vi "FlowSensorSampleSensorLoop.vi"   [LabVIEW 2018]
uses:
  FlowSensorSampleSensorLoopData.ctl
  FlowSensorSampleSensorLoopStates.ctl
  FlowSensorSample.ctl
  FlowSensorErrorSample.ctl
  FlowSensorErrorCodes.ctl
  <vilib>/Platform/TimedLoop/XDataNode/timing_clust.ctl
  <vilib>/Platform/TimedLoop/XDataNode/nitl_modes.ctl
  <vilib>/Platform/TimedLoop/XDataNode/wakeup.ctl
  <vilib>/rvi/Emulation/niFpgaSctlEmulationGetInTimedLoop.vi
  <vilib>/rvi/Emulation/niFpgaEmulationReportErrorSimple.vi
  <vilib>/rvi/Emulation/niFpgaGetClockAttributes.vi
  <vilib>/rvi/Emulation/niFpgaCriticalErrorInLSC.vi
  <vilib>/rvi/Emulation/niFpgaEmulationIsFPGAContextNoSignature.vi
  <vilib>/rvi/errors/niFpgaSetErrorForExecOnDevCompSimple.vi
  <vilib>/rvi/eio/common/nirviEmuReportErrorAndStop.vi
  <vilib>/rvi/DataTransferAndStorage/Container/Common/niFpgaContainerGetUniqueNameForEmu.vi
  <vilib>/rvi/FIFO/Fifo_Resource/nirvififoEmulationSetSize.vi
  <vilib>/rvi/FIFO/Fifo_Resource/nirviFifoEmulationQueueMgr.vi
  <instcachedir>/0/nirviFifoEmulationQueueMgr_E5CAEC123FF24DC58D834DCA3CDAA9B5.lvgen/nirviFifoEmulationQueueMgr_E5CAEC123FF24DC58D834DCA3CDAA9B5_002.vi
  <vilib>/Utility/error.llb/Clear Errors.vi
  <vilib>/rvi/FIFO/Fifo_Resource/nirvififoEmulationCreateLock.vi
  <vilib>/rvi/Emulation/niFpgaProcessEmulError.vi
  <vilib>/rvi/FIFO/Fifo_Resource/nirvififoEmulationObtainLock.vi
  <vilib>/rvi/FIFO/Fifo_Resource/nirvififoEmulationReleaseLock.vi
  <vilib>/rvi/occurrence/nirviWaitOnOccurrenceBase.vi
  <vilib>/rvi/errors/nirviReportUnexpectedCaseInternalError.vi
  <vilib>/rvi/errors/nirviReportUnexpectedCaseInternalError (U32).vi
  <vilib>/rvi/FIFO/Fifo_Resource/nirvififoEmulationDetermineInputValidOut.vi
  <instcachedir>/0/nirviFifoEmulationQueueMgr_E5CAEC123FF24DC58D834DCA3CDAA9B5.lvgen/nirviFifoEmulationQueueMgr_E5CAEC123FF24DC58D834DCA3CDAA9B5_001.vi
  <instcachedir>/0/nirviFifoEmulationQueueMgr_E5CAEC123FF24DC58D834DCA3CDAA9B5.lvgen/nirviFifoEmulationQueueMgr_E5CAEC123FF24DC58D834DCA3CDAA9B5_004.vi
  <vilib>/rvi/Memory/Memory_Emulation/niFpgaMemoryEmulationCacheClearOnFirstRun.vi
  <vilib>/rvi/Memory/Memory_Emulation/nirvimemoryEmulationManagerCache_MakeExclusive.vi
  <vilib>/rvi/Memory/Memory_Emulation/niFpgaMemoryEmulationValidateCache.vi
  <vilib>/rvi/Memory/Memory_Emulation/nirvimemoryEmulationManagerCache_InsertValue.vi
  <vilib>/rvi/Memory/Memory_Emulation/nirvimemoryEmulationManagerCache_ReleaseExclusive.vi
  <vilib>/rvi/Memory/Memory_Emulation/nirvimemoryEmulationManagerCache_GetValue.vi
  <vilib>/rvi/Memory/Memory_Emulation/nirvimemoryEmulationManagerCache_SetValue.vi
  <instcachedir>/0/nirviFifoEmulationQueueMgr_E5CAEC123FF24DC58D834DCA3CDAA9B5.lvgen/nirviFifoEmulationQueueMgr_E5CAEC123FF24DC58D834DCA3CDAA9B5_028.vi
  <instcachedir>/0/nirviFifoEmulationQueueMgr_E5CAEC123FF24DC58D834DCA3CDAA9B5.lvgen/nirviFifoEmulationQueueMgr_E5CAEC123FF24DC58D834DCA3CDAA9B5_015.vi
  <vilib>/Platform/TimedLoop/XDataNode/XDataNode.xnode
  <vilib>/rvi/DataTransferAndStorage/Container/XNode/niFpgaContainer.xnode
  <vilib>/rvi/FIFO/Fifo_Resource/nirvififoEmulationRead.vi
  <vilib>/rvi/FIFO/Fifo_Resource/nirvififoEmulationWrite.vi
  <vilib>/rvi/DataTransferAndStorage/Register/Emulation/niFpgaRegisterEmulation.vi
  <vilib>/Platform/TimedLoop/XDataNode/XDNodeRunTimeDep.lvlib
types:
  T1 = typedef "FlowSensorSampleSensorLoopData.ctl" = cluster{"State":T2, "StateAfterRead":T2, "Timestamp":u64, "Timeout":i32, "U32":u32, "CRC":u16, "Exception":u8, "Sample":T3, "ErrorSample":T4}
  T2 = typedef "FlowSensorSampleSensorLoopStates.ctl" = enum16{"WaitForTrigger", "ClearRxFIFO", "WaitForClearComplete", "WriteAddress", "WriteFunction", "WriteStartAddress1", "WriteStartAddress0", "WriteAddressCount1", "WriteAddressCount0", "WriteCRC1", "WriteCRC0", "ReadAddress", "ReadFunction", "ReadByteCount", "StartSignalStrength", "EndSignalStrength", "StartFlowRate", "EndFlowRate", "StartNetTotalizer", "EndNetTotalizer", "StartPositiveTotalizer", "EndPositiveTotalizer", "StartNegativeTotalizer", "EndNegativeTotalizer", "StartTemperature1", "EndTemperature1", "StartTemperature2", "EndTemperature2", "ReadDataByte1", "ReadDataByte0", "ReadDataByte3", "ReadDataByte2", "ReadCRCByte0", "ReadCRCByte1", "CalculateCRC", "ValidateCRC", "PrepareSample", "MoveSample", "ReadExceptionCode", "ReadExceptionCRCByte0", "ReadExceptionCRCByte1", "CalculateExceptionCRC", "ValidateExceptionCRC", "ParseExceptionCode", "ResponseAddressError", "ResponseFunctionCodeError", "ResponseByteCountError", "ResponseCRCError", "ResponseUnknownError", "ResponseTimeoutError", "SensorReportsIllegalFunction", "SensorReportsIllegalDataAddress", "PrepareErrorCode", "MoveErrorCode"}
  T3 = typedef "FlowSensorSample.ctl" = cluster{"Timestamp":u64, "TxBytes":u64, "RxBytes":u64, "TxFrames":u64, "RxFrames":u64, "SignalStrength":u32, "FlowRate":u32, "NetTotalizer":u32, "PositiveTotalizer":u32, "NegativeTotalizer":u32, "Temperature1":u32, "Temperature2":u32}
  T4 = typedef "FlowSensorErrorSample.ctl" = cluster{"Timestamp":u64, "TxBytes":u64, "RxBytes":u64, "TxFrames":u64, "RxFrames":u64, "ErrorCode":T5}
  T5 = typedef "FlowSensorErrorCodes.ctl" = enum8{"None", "ResponseAddressError", "ResponseFunctionCodeError", "ResponseByteCountError", "ResponseCRCError", "ResponseUnknownError", "ResponseTimeoutError", "SensorReportsIllegalFunction", "SensorReportsIllegalDataAddress"}
  T6 = typedef "XDNodeRunTimeDep.lvlib/timing_clust.ctl" = cluster{"Expected End [f-1]":u64, "Actual End [f-1]":u64, "Finished Late? [f-1]":bool, "Expected End [i-1]":u64, "Actual End [i-1]":u64, "Finished Late? [i-1]":bool, "Expected Start [i]":u64, "Actual Start [i]":u64, "Expected Start [f]":u64, "Actual Start [f]":u64, "Source Name":string, "Structure Name":string, "Period":i64, "Deadline":i64, "Offset":i64, "Start":i64, "Priority":i32, "Timeout":i32, "Mode":T7, "Wakeup Reason":T8, "Error":errorcluster, "Source Type":string, "Secondary Source Type":string, "Global End Time":u64, "Global Start Time":u64, "Frame Duration":u64, "Iteration Duration":u64, "Assigned CPU":i32, "I/O Scan Engine Mode":u32}
  T7 = typedef "XDNodeRunTimeDep.lvlib/nitl_modes.ctl" = enum32{"No Change", "Process missed periods, maintain original phase", "Discard missed periods, maintain original phase", "Process missed periods, ignore original phase", "Discard missed periods, ignore original phase"}
  T8 = typedef "XDNodeRunTimeDep.lvlib/wakeup.ctl" = enum32{"Normal", "Aborted", "Asynchronous wakeup", "Timing source error", "Timed loop error", "Timeout"}
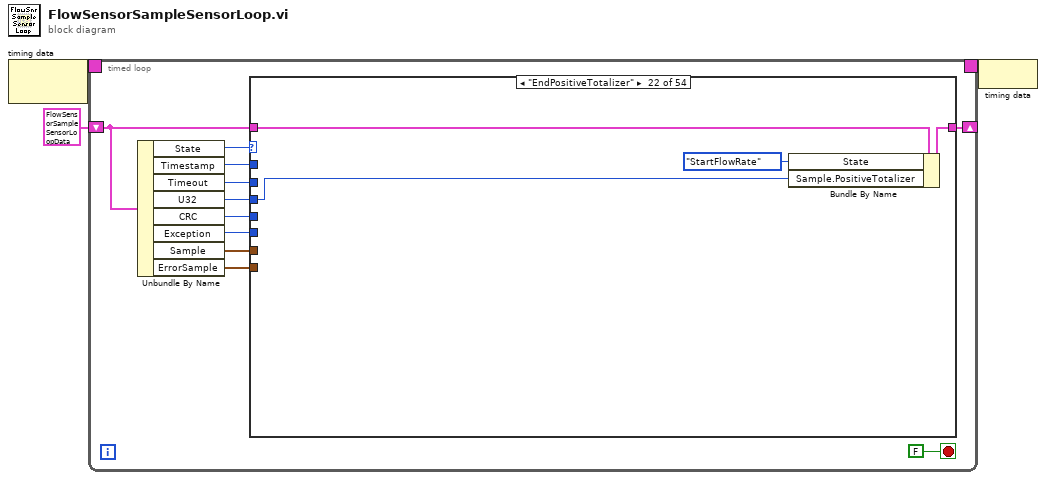
[diagram p0: block diagram]
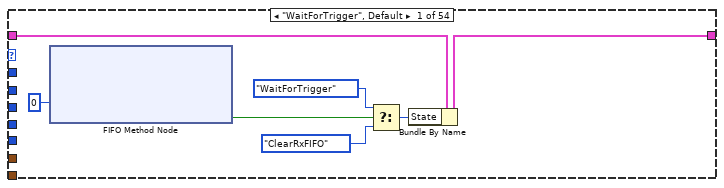
[diagram p2: hidden frame]
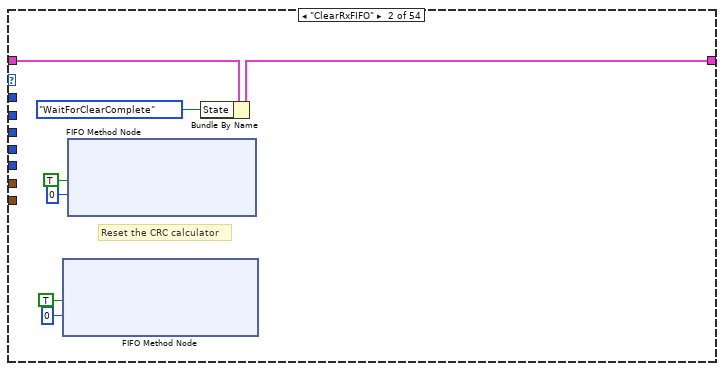
[diagram p3: hidden frame]
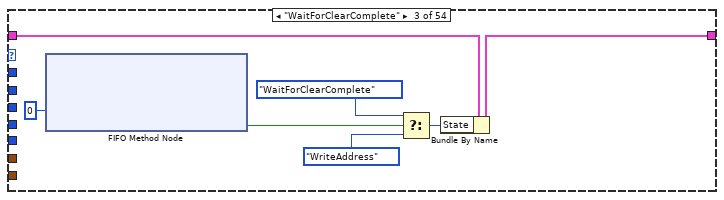
[diagram p4: hidden frame]
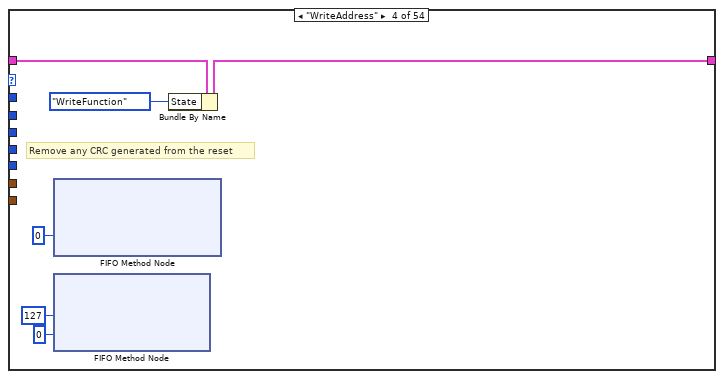
[diagram p5: hidden frame]
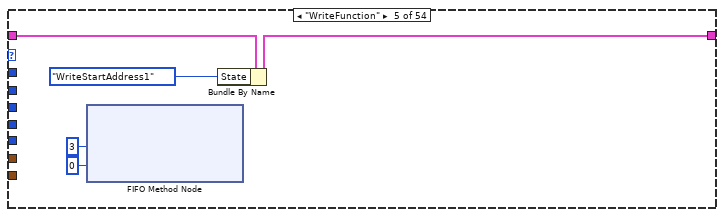
[diagram p6: hidden frame]
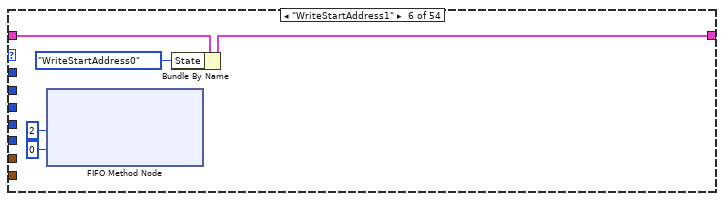
[diagram p7: hidden frame]
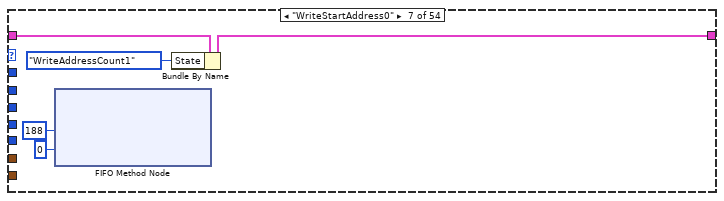
[diagram p8: hidden frame]
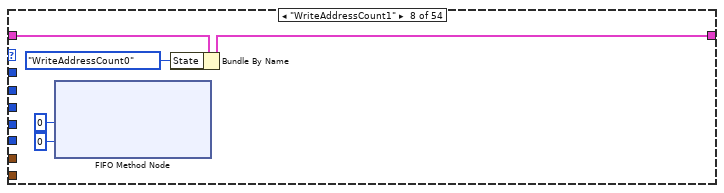
[diagram p9: hidden frame]
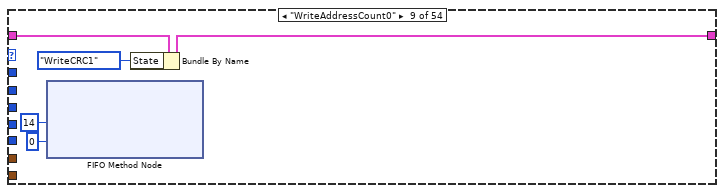
[diagram p10: hidden frame]
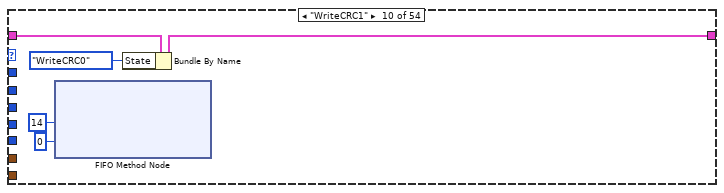
[diagram p11: hidden frame]
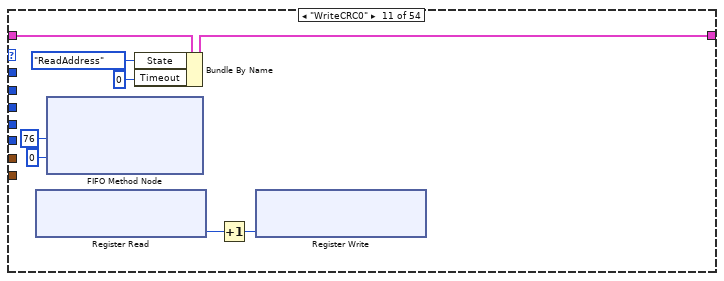
[diagram p12: hidden frame]
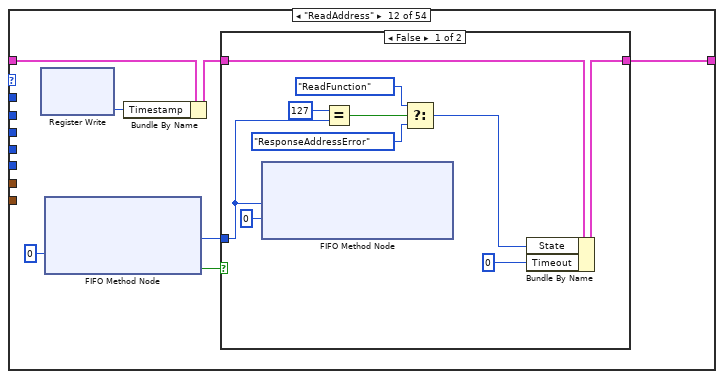
[diagram p13: hidden frame]
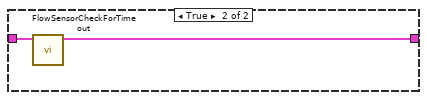
[diagram p14: hidden frame]
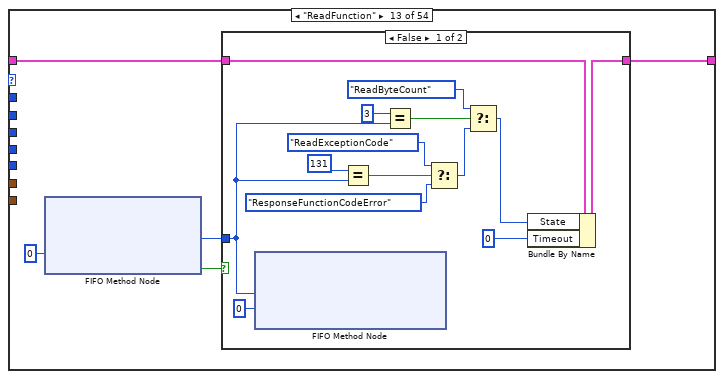
[diagram p15: hidden frame]
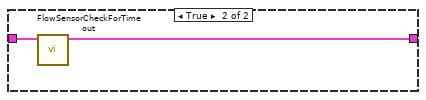
[diagram p16: hidden frame]
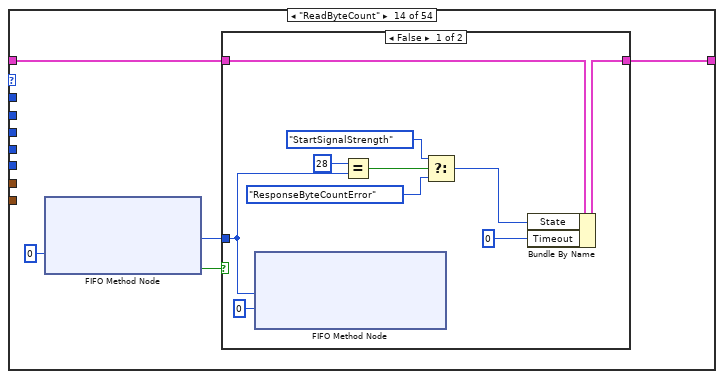
[diagram p17: hidden frame]
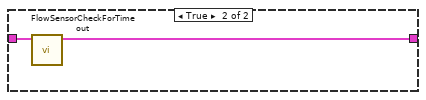
[diagram p18: hidden frame]
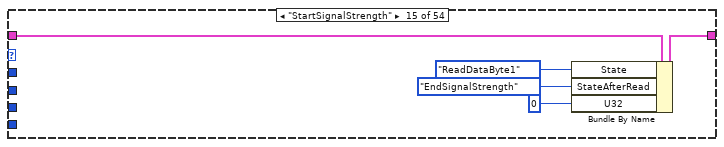
[diagram p19: hidden frame]
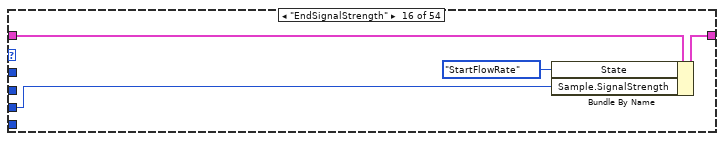
[diagram p20: hidden frame]
diagram:
  n1 = node-c288() -> (w3:T6)  [unwired: 1 in]
  n2 = timed-loop {
    timing: w3 -> [_]
    timing-out: [_] -> w2
    shift-right: [w13] -> _
    shift-left: T1 {"State"=enum."WaitForTrigger", "StateAfterRead"=enum."ClearRxFIFO", "Timestamp"=0, "Timeout"=0, "U32"=0, "CRC"=0, "Exception"=0, "Sample"={"Timestamp"=0, "TxBytes"=0, "RxBytes"=0, "TxFrames"=0, "RxFrames"=0, "SignalStrength"=0, "FlowRate"=0, "NetTotalizer"=0, "PositiveTotalizer"=0, "NegativeTotalizer"=0, "Temperature1"=0, "Temperature2"=0}, "ErrorSample"={"Timestamp"=0, "TxBytes"=0, "RxBytes"=0, "TxFrames"=0, "RxFrames"=0, "ErrorCode"=enum."None"}} ("InclinometerData") -> [w14]
    stop <- FALSE stop-if-true
    n3 = Unbundle By Name(w14) -> ("State"=w12:T2, "Timestamp"=w7:u64, "Timeout"=w11:i32, "U32"=w10:u32, "CRC"=w9:u16, "Exception"=w6:u8, "Sample"=w5:T3, "ErrorSample"=w4:T4)
    n4 = case shown="\"EndPositiveTotalizer\"" w12 {
      tunnel: w14 -> [w20 w27 w34 w40 w45 w50 w55 w60 w65 w70 w78 w82 w99 w120 w141 w145 w150 w154 w159 w163 w168 w172 w177 w181 w186 w190 w195 w199 w201 w224 w245 w266 w287 w307 w327 w332 w352 w357 w361 w382 w402 w422 w427 w447 w451 w455 w459 w463 w467 w471 w475 w479 w487 w492]
      tunnel: [w21 w28 w35 w41 w46 w51 w56 w61 w66 w71 w79 w83 w100 w121 w140 w144 w149 w153 w158 w162 w167 w171 w176 w180 w185 w189 w194 w198 w202 w225 w246 w267 w288 w308 w328 w333 w353 w358 w362 w383 w403 w423 w428 w448 w452 w456 w460 w464 w468 w472 w476 w480 w488 w493] -> w13
      tunnel: w11 -> [_ _ _ _ _ _ _ _ _ _ _ _ _ _ _ _ _ _ _ _ _ _ _ _ _ _ _ _ _ _ _ _ _ _ _ _ _ _ _ _ _ _ _ _ _ _ _ _ _ _ _ _ _ _]
      tunnel: w10 -> [_ _ _ _ _ _ _ _ _ _ _ _ _ _ _ w142 _ w151 _ w160 _ w169 _ w178 _ w187 _ w196 w200 w223 w244 w265 _ _ _ _ _ _ _ _ _ _ _ _ _ _ _ _ _ _ _ _ _ _]
      tunnel: w9 -> [_ _ _ _ _ _ _ _ _ _ _ _ _ _ _ _ _ _ _ _ _ _ _ _ _ _ _ _ _ _ _ _ w286 w306 _ w331 _ _ _ w381 w401 _ w426 _ _ _ _ _ _ _ _ _ _ _]
      tunnel: w7 -> [_ _ _ _ _ _ _ _ _ _ _ _ _ _ _ _ _ _ _ _ _ _ _ _ _ _ _ _ _ _ _ _ _ _ _ _ w351 _ _ _ _ _ _ _ _ _ _ _ _ _ _ _ w486 _]
      tunnel: w6 -> [_ _ _ _ _ _ _ _ _ _ _ _ _ _ _ _ _ _ _ _ _ _ _ _ _ _ _ _ _ _ _ _ _ _ _ _ _ _ _ _ _ _ _ w442 _ _ _ _ _ _ _ _ _ _]
      tunnel: w5 -> [_ _ _ _ _ _ _ _ _ _ _ _ _ _ _ _ _ _ _ _ _ _ _ _ _ _ _ _ _ _ _ _ _ _ _ _ _ w354 _ _ _ _ _ _ _ _ _ _ _ _ _ _ _ _]
      tunnel: w4 -> [_ _ _ _ _ _ _ _ _ _ _ _ _ _ _ _ _ _ _ _ _ _ _ _ _ _ _ _ _ _ _ _ _ _ _ _ _ _ _ _ _ _ _ _ _ _ _ _ _ _ _ _ _ w490]
      frame "WaitForTrigger", Default {
        n5 = xnode ("FIFO Method Node")("Timeout"=0) -> ("Timed Out?"=w15:bool)  [unwired: 1 in, 2 out]
        n6 = Select(t=FlowSensorSampleSensorLoopStates."WaitForTrigger" ("InclinometerState"), s=w15, f=FlowSensorSampleSensorLoopStates."ClearRxFIFO" ("InclinometerState")) -> (s? t:f=w17:T2)
        n7 = Bundle By Name(cluster=w20, "State"=w17) -> (w21:T1)
      }
      frame "ClearRxFIFO" {
        # "Reset the CRC calculator"
        n8 = xnode ("FIFO Method Node")("Element"=TRUE, "Timeout"=0) -> ()  [unwired: 1 in, 2 out]
        n9 = xnode ("FIFO Method Node")("Element"=TRUE, "Timeout"=0) -> ()  [unwired: 1 in, 2 out]
        n10 = Bundle By Name(cluster=w27, "State"=FlowSensorSampleSensorLoopStates."WaitForClearComplete" ("InclinometerState")) -> (w28:T1)
      }
      frame "WaitForClearComplete" {
        n11 = xnode ("FIFO Method Node")("Timeout"=0) -> ("Timed Out?"=w29:bool)  [unwired: 1 in, 2 out]
        n12 = Select(t=FlowSensorSampleSensorLoopStates."WaitForClearComplete", s=w29, f=FlowSensorSampleSensorLoopStates."WriteAddress" ("InclinometerState")) -> (s? t:f=w31:T2)
        n13 = Bundle By Name(cluster=w34, "State"=w31) -> (w35:T1)
      }
      frame "WriteAddress" {
        # "Remove any CRC generated from the reset"
        n14 = xnode ("FIFO Method Node")("Timeout"=0) -> ()  [unwired: 1 in, 3 out]
        n15 = xnode ("FIFO Method Node")("Element"=u8 127, "Timeout"=0) -> ()  [unwired: 1 in, 2 out]
        n16 = Bundle By Name(cluster=w40, "State"=FlowSensorSampleSensorLoopStates."WriteFunction" ("InclinometerState")) -> (w41:T1)
      }
      frame "WriteFunction" {
        n17 = xnode ("FIFO Method Node")("Element"=u8 3, "Timeout"=0) -> ()  [unwired: 1 in, 2 out]
        n18 = Bundle By Name(cluster=w45, "State"=FlowSensorSampleSensorLoopStates."WriteStartAddress1" ("InclinometerState")) -> (w46:T1)
      }
      frame "WriteStartAddress1" {
        n19 = xnode ("FIFO Method Node")("Element"=u8 2, "Timeout"=0) -> ()  [unwired: 1 in, 2 out]
        n20 = Bundle By Name(cluster=w50, "State"=FlowSensorSampleSensorLoopStates."WriteStartAddress0" ("InclinometerState")) -> (w51:T1)
      }
      frame "WriteStartAddress0" {
        n21 = xnode ("FIFO Method Node")("Element"=u8 188, "Timeout"=0) -> ()  [unwired: 1 in, 2 out]
        n22 = Bundle By Name(cluster=w55, "State"=FlowSensorSampleSensorLoopStates."WriteAddressCount1" ("InclinometerState")) -> (w56:T1)
      }
      frame "WriteAddressCount1" {
        n23 = xnode ("FIFO Method Node")("Element"=u8 0, "Timeout"=0) -> ()  [unwired: 1 in, 2 out]
        n24 = Bundle By Name(cluster=w60, "State"=FlowSensorSampleSensorLoopStates."WriteAddressCount0" ("InclinometerState")) -> (w61:T1)
      }
      frame "WriteAddressCount0" {
        n25 = xnode ("FIFO Method Node")("Element"=u8 14, "Timeout"=0) -> ()  [unwired: 1 in, 2 out]
        n26 = Bundle By Name(cluster=w65, "State"=FlowSensorSampleSensorLoopStates."WriteCRC1" ("InclinometerState")) -> (w66:T1)
      }
      frame "WriteCRC1" {
        n27 = xnode ("FIFO Method Node")("Element"=u8 14, "Timeout"=0) -> ()  [unwired: 1 in, 2 out]
        n28 = Bundle By Name(cluster=w70, "State"=FlowSensorSampleSensorLoopStates."WriteCRC0" ("InclinometerState")) -> (w71:T1)
      }
      frame "WriteCRC0" {
        n29 = xnode ("Register Read")() -> ("Data"=w73:u64)  [unwired: 1 in, 1 out]
        n30 = xnode ("FIFO Method Node")("Element"=u8 76, "Timeout"=0) -> ()  [unwired: 1 in, 2 out]
        n31 = Bundle By Name(cluster=w78, "State"=FlowSensorSampleSensorLoopStates."ReadAddress" ("InclinometerState"), "Timeout"=0) -> (w79:T1)
        n32 = Increment(x=w73) -> (x+1=w72:u64)
        n33 = xnode ("Register Write")("Data"=w72) -> ()  [unwired: 1 in, 1 out]
      }
      frame "ReadAddress" {
        n34 = xnode "Register Write"() -> ("Data"=w80:u64)  [unwired: 1 in, 1 out]
        n35 = xnode ("FIFO Method Node")("Timeout"=0) -> ("Element"=w84:u8, "Timed Out?"=w85:bool)  [unwired: 1 in, 1 out]
        n36 = Bundle By Name(cluster=w82, "Timestamp"=w80) -> (w81:T1)
        n37 = case shown="False" w85 {
          tunnel: w84 -> [w93 _]
          tunnel: [w95 w97] -> w83
          tunnel: w81 -> [w96 w98]
          frame False {
            n38 = xnode ("FIFO Method Node")("Element"=w93, "Timeout"=0) -> ()  [unwired: 1 in, 2 out]
            n39 = Equal?(x=u8 127, y=w93) -> (x = y?=w91:bool)
            n40 = Select(t=FlowSensorSampleSensorLoopStates."ReadFunction" ("InclinometerState"), s=w91, f=FlowSensorSampleSensorLoopStates."ResponseAddressError" ("InclinometerState")) -> (s? t:f=w88:T2)
            n41 = Bundle By Name(cluster=w96, "State"=w88, "Timeout"=0) -> (w95:T1)
          }
          frame True {
            n42 = call "FlowSensorCheckForTimeout.vi"("FlowSensorSampleSensorLoopData in"=w98) -> ("FlowSensorSampleSensorLoopData out"=w97:T1)  [unwired: 10 in]
          }
        }
      }
      frame "ReadFunction" {
        n43 = xnode ("FIFO Method Node")("Timeout"=0) -> ("Element"=w101:u8, "Timed Out?"=w102:bool)  [unwired: 1 in, 1 out]
        n44 = case shown="False" w102 {
          tunnel: w101 -> [w109 _]
          tunnel: [w116 w118] -> w100
          tunnel: w99 -> [w117 w119]
          frame False {
            n45 = xnode ("FIFO Method Node")("Element"=w109, "Timeout"=0) -> ()  [unwired: 1 in, 2 out]
            n46 = Equal?(x=u8 131, y=w109) -> (x = y?=w108:bool)
            n47 = Equal?(x=u8 3, y=w109) -> (x = y?=w113:bool)
            n48 = Select(t=FlowSensorSampleSensorLoopStates."ReadExceptionCode" ("InclinometerState"), s=w108, f=FlowSensorSampleSensorLoopStates."ResponseFunctionCodeError" ("InclinometerState")) -> (s? t:f=w111:T2)
            n49 = Select(t=FlowSensorSampleSensorLoopStates."ReadByteCount" ("InclinometerState"), s=w113, f=w111) -> (s? t:f=w105:T2)
            n50 = Bundle By Name(cluster=w117, "State"=w105, "Timeout"=0) -> (w116:T1)
          }
          frame True {
            n51 = call "FlowSensorCheckForTimeout.vi"("FlowSensorSampleSensorLoopData in"=w119) -> ("FlowSensorSampleSensorLoopData out"=w118:T1)  [unwired: 10 in]
          }
        }
      }
      frame "ReadByteCount" {
        n52 = xnode ("FIFO Method Node")("Timeout"=0) -> ("Element"=w122:u8, "Timed Out?"=w123:bool)  [unwired: 1 in, 1 out]
        n53 = case shown="False" w123 {
          tunnel: w122 -> [w131 _]
          tunnel: [w133 w135] -> w121
          tunnel: w120 -> [w134 w136]
          frame False {
            n54 = xnode ("FIFO Method Node")("Element"=w131, "Timeout"=0) -> ()  [unwired: 1 in, 2 out]
            n55 = Equal?(x=u8 28, y=w131) -> (x = y?=w129:bool)
            n56 = Select(t=FlowSensorSampleSensorLoopStates."StartSignalStrength" ("InclinometerState"), s=w129, f=FlowSensorSampleSensorLoopStates."ResponseByteCountError" ("InclinometerState")) -> (s? t:f=w126:T2)
            n57 = Bundle By Name(cluster=w134, "State"=w126, "Timeout"=0) -> (w133:T1)
          }
          frame True {
            n58 = call "FlowSensorCheckForTimeout.vi"("FlowSensorSampleSensorLoopData in"=w136) -> ("FlowSensorSampleSensorLoopData out"=w135:T1)  [unwired: 10 in]
          }
        }
      }
      frame "StartSignalStrength" {
        n59 = Bundle By Name(cluster=w141, "State"=FlowSensorSampleSensorLoopStates."ReadDataByte1", "StateAfterRead"=FlowSensorSampleSensorLoopStates."EndSignalStrength", "U32"=u32 0) -> (w140:T1)
      }
      frame "EndSignalStrength" {
        n60 = Bundle By Name(cluster=w145, "State"=FlowSensorSampleSensorLoopStates."StartFlowRate", "Sample.SignalStrength"=w142) -> (w144:T1)
      }
      frame "StartFlowRate" {
        n61 = Bundle By Name(cluster=w150, "State"=FlowSensorSampleSensorLoopStates."ReadDataByte1", "StateAfterRead"=FlowSensorSampleSensorLoopStates."EndFlowRate", "U32"=u32 0) -> (w149:T1)
      }
      frame "EndFlowRate" {
        n62 = Bundle By Name(cluster=w154, "State"=FlowSensorSampleSensorLoopStates."StartNetTotalizer", "Sample.FlowRate"=w151) -> (w153:T1)
      }
      frame "StartNetTotalizer" {
        n63 = Bundle By Name(cluster=w159, "State"=FlowSensorSampleSensorLoopStates."ReadDataByte1", "StateAfterRead"=FlowSensorSampleSensorLoopStates."EndNetTotalizer", "U32"=u32 0) -> (w158:T1)
      }
      frame "EndNetTotalizer" {
        n64 = Bundle By Name(cluster=w163, "State"=FlowSensorSampleSensorLoopStates."StartPositiveTotalizer", "Sample.NetTotalizer"=w160) -> (w162:T1)
      }
      frame "StartPositiveTotalizer" {
        n65 = Bundle By Name(cluster=w168, "State"=FlowSensorSampleSensorLoopStates."ReadDataByte1", "StateAfterRead"=FlowSensorSampleSensorLoopStates."EndPositiveTotalizer", "U32"=u32 0) -> (w167:T1)
      }
      frame "EndPositiveTotalizer" {
        n66 = Bundle By Name(cluster=w172, "State"=FlowSensorSampleSensorLoopStates."StartFlowRate", "Sample.PositiveTotalizer"=w169) -> (w171:T1)
      }
      frame "StartNegativeTotalizer" {
        n67 = Bundle By Name(cluster=w177, "State"=FlowSensorSampleSensorLoopStates."ReadDataByte1", "StateAfterRead"=FlowSensorSampleSensorLoopStates."EndNegativeTotalizer", "U32"=u32 0) -> (w176:T1)
      }
      frame "EndNegativeTotalizer" {
        n68 = Bundle By Name(cluster=w181, "State"=FlowSensorSampleSensorLoopStates."StartTemperature1", "Sample.NegativeTotalizer"=w178) -> (w180:T1)
      }
      frame "StartTemperature1" {
        n69 = Bundle By Name(cluster=w186, "State"=FlowSensorSampleSensorLoopStates."ReadDataByte1", "StateAfterRead"=FlowSensorSampleSensorLoopStates."EndTemperature1", "U32"=u32 0) -> (w185:T1)
      }
      frame "EndTemperature1" {
        n70 = Bundle By Name(cluster=w190, "State"=FlowSensorSampleSensorLoopStates."StartTemperature2", "Sample.Temperature1"=w187) -> (w189:T1)
      }
      frame "StartTemperature2" {
        n71 = Bundle By Name(cluster=w195, "State"=FlowSensorSampleSensorLoopStates."ReadDataByte1", "StateAfterRead"=FlowSensorSampleSensorLoopStates."EndTemperature2", "U32"=u32 0) -> (w194:T1)
      }
      frame "EndTemperature2" {
        n72 = Bundle By Name(cluster=w199, "State"=FlowSensorSampleSensorLoopStates."ReadCRCByte0", "Sample.Temperature2"=w196) -> (w198:T1)
      }
      frame "ReadDataByte1" {
        n73 = xnode ("FIFO Method Node")("Timeout"=0) -> ("Element"=w203:u8, "Timed Out?"=w204:bool)  [unwired: 1 in, 1 out]
        n74 = case shown="False" w204 {
          tunnel: w203 -> [w209 _]
          tunnel: [w217 w219] -> w202
          tunnel: w201 -> [w218 w220]
          tunnel: w200 -> [w213 _]
          frame False {
            n75 = To Unsigned Long Integer(number=w209) -> (unsigned 32bit integer=w208:u32)
            n76 = xnode ("FIFO Method Node")("Element"=w209, "Timeout"=0) -> ()  [unwired: 1 in, 2 out]
            n77 = Logical Shift(y=i16 8, x=w208) -> (x << y=w211:u32)
            n78 = And(x=u32 4294902015, y=w213) -> (x .and. y?=w210:u32)
            n79 = Or(x=w210, y=w211) -> (x .or. y?=w207:u32)
            n80 = Bundle By Name(cluster=w218, "State"=FlowSensorSampleSensorLoopStates."ReadDataByte0" ("InclinometerState"), "U32"=w207, "Timeout"=0) -> (w217:T1)
          }
          frame True {
            n81 = call "FlowSensorCheckForTimeout.vi"("FlowSensorSampleSensorLoopData in"=w220) -> ("FlowSensorSampleSensorLoopData out"=w219:T1)  [unwired: 10 in]
          }
        }
      }
      frame "ReadDataByte0" {
        n82 = xnode ("FIFO Method Node")("Timeout"=0) -> ("Element"=w226:u8, "Timed Out?"=w222:bool)  [unwired: 1 in, 1 out]
        n83 = case shown="False" w222 {
          tunnel: w226 -> [w227 _]
          tunnel: [w238 w240] -> w225
          tunnel: w224 -> [w239 w241]
          tunnel: w223 -> [w235 _]
          frame False {
            n84 = To Unsigned Long Integer(number=w227) -> (unsigned 32bit integer=w231:u32)
            n85 = xnode ("FIFO Method Node")("Element"=w227, "Timeout"=0) -> ()  [unwired: 1 in, 2 out]
            n86 = Logical Shift(y=i16 0, x=w231) -> (x << y=w233:u32)
            n87 = And(x=u32 4294967040, y=w235) -> (x .and. y?=w232:u32)
            n88 = Or(x=w232, y=w233) -> (x .or. y?=w230:u32)
            n89 = Bundle By Name(cluster=w239, "State"=FlowSensorSampleSensorLoopStates."ReadDataByte3" ("InclinometerState"), "U32"=w230, "Timeout"=0) -> (w238:T1)
          }
          frame True {
            n90 = call "FlowSensorCheckForTimeout.vi"("FlowSensorSampleSensorLoopData in"=w241) -> ("FlowSensorSampleSensorLoopData out"=w240:T1)  [unwired: 10 in]
          }
        }
      }
      frame "ReadDataByte3" {
        n91 = xnode ("FIFO Method Node")("Timeout"=0) -> ("Element"=w247:u8, "Timed Out?"=w242:bool)  [unwired: 1 in, 1 out]
        n92 = case shown="False" w242 {
          tunnel: w247 -> [w249 _]
          tunnel: [w259 w261] -> w246
          tunnel: w245 -> [w260 w262]
          tunnel: w244 -> [w256 _]
          frame False {
            n93 = To Unsigned Long Integer(number=w249) -> (unsigned 32bit integer=w252:u32)
            n94 = xnode ("FIFO Method Node")("Element"=w249, "Timeout"=0) -> ()  [unwired: 1 in, 2 out]
            n95 = Logical Shift(y=i16 24, x=w252) -> (x << y=w254:u32)
            n96 = And(x=u32 16777215, y=w256) -> (x .and. y?=w253:u32)
            n97 = Or(x=w253, y=w254) -> (x .or. y?=w251:u32)
            n98 = Bundle By Name(cluster=w260, "State"=FlowSensorSampleSensorLoopStates."ReadDataByte2" ("InclinometerState"), "U32"=w251, "Timeout"=0) -> (w259:T1)
          }
          frame True {
            n99 = call "FlowSensorCheckForTimeout.vi"("FlowSensorSampleSensorLoopData in"=w262) -> ("FlowSensorSampleSensorLoopData out"=w261:T1)  [unwired: 10 in]
          }
        }
      }
      frame "ReadDataByte2" {
        n100 = xnode ("FIFO Method Node")("Timeout"=0) -> ("Element"=w268:u8, "Timed Out?"=w263:bool)  [unwired: 1 in, 1 out]
        n101 = case shown="False" w263 {
          tunnel: w268 -> [w271 _]
          tunnel: [w281 w282] -> w267
          tunnel: w266 -> [w270 w283]
          tunnel: w265 -> [w279 _]
          frame False {
            n102 = To Unsigned Long Integer(number=w271) -> (unsigned 32bit integer=w275:u32)
            n103 = xnode ("FIFO Method Node")("Element"=w271, "Timeout"=0) -> ()  [unwired: 1 in, 2 out]
            n104 = Logical Shift(y=i16 16, x=w275) -> (x << y=w277:u32)
            n105 = And(x=u32 4278255615, y=w279) -> (x .and. y?=w276:u32)
            n106 = Or(x=w276, y=w277) -> (x .or. y?=w274:u32)
            n107 = Unbundle By Name(w270) -> ("StateAfterRead"=w269:T2)
            n108 = Bundle By Name(cluster=w270, "State"=w269, "U32"=w274, "Timeout"=0) -> (w281:T1)
          }
          frame True {
            n109 = call "FlowSensorCheckForTimeout.vi"("FlowSensorSampleSensorLoopData in"=w283) -> ("FlowSensorSampleSensorLoopData out"=w282:T1)  [unwired: 10 in]
          }
        }
      }
      frame "ReadCRCByte0" {
        n110 = xnode ("FIFO Method Node")("Timeout"=0) -> ("Element"=w289:u8, "Timed Out?"=w284:bool)  [unwired: 1 in, 1 out]
        n111 = case shown="False" w284 {
          tunnel: w289 -> [w290 _]
          tunnel: [w300 w302] -> w288
          tunnel: w287 -> [w301 w303]
          tunnel: w286 -> [w292 _]
          frame False {
            n112 = To Unsigned Word Integer(number=w290) -> (unsigned 16bit integer=w294:u16)
            n113 = Logical Shift(y=i16 0, x=w294) -> (x << y=w296:u16)
            n114 = And(x=u16 65280, y=w292) -> (x .and. y?=w295:u16)
            n115 = Or(x=w295, y=w296) -> (x .or. y?=w293:u16)
            n116 = Bundle By Name(cluster=w301, "State"=FlowSensorSampleSensorLoopStates."ReadCRCByte1" ("InclinometerState"), "CRC"=w293, "Timeout"=0) -> (w300:T1)
          }
          frame True {
            n117 = call "FlowSensorCheckForTimeout.vi"("FlowSensorSampleSensorLoopData in"=w303) -> ("FlowSensorSampleSensorLoopData out"=w302:T1)  [unwired: 10 in]
          }
        }
      }
      frame "ReadCRCByte1" {
        n118 = xnode ("FIFO Method Node")("Timeout"=0) -> ("Element"=w309:u8, "Timed Out?"=w304:bool)  [unwired: 1 in, 1 out]
        n119 = case shown="False" w304 {
          tunnel: w309 -> [w310 _]
          tunnel: [w320 w322] -> w308
          tunnel: w307 -> [w321 w323]
          tunnel: w306 -> [w312 _]
          frame False {
            n120 = To Unsigned Word Integer(number=w310) -> (unsigned 16bit integer=w314:u16)
            n121 = Logical Shift(y=i16 8, x=w314) -> (x << y=w316:u16)
            n122 = And(x=u16 255, y=w312) -> (x .and. y?=w315:u16)
            n123 = Or(x=w315, y=w316) -> (x .or. y?=w313:u16)
            n124 = Bundle By Name(cluster=w321, "State"=FlowSensorSampleSensorLoopStates."CalculateCRC" ("InclinometerState"), "CRC"=w313, "Timeout"=0) -> (w320:T1)
          }
          frame True {
            n125 = call "FlowSensorCheckForTimeout.vi"("FlowSensorSampleSensorLoopData in"=w323) -> ("FlowSensorSampleSensorLoopData out"=w322:T1)  [unwired: 10 in]
          }
        }
      }
      frame "CalculateCRC" {
        n126 = xnode ("FIFO Method Node")("Element"=TRUE, "Timeout"=0) -> ()  [unwired: 1 in, 2 out]
        n127 = Bundle By Name(cluster=w327, "State"=FlowSensorSampleSensorLoopStates."ValidateCRC" ("InclinometerState")) -> (w328:T1)
      }
      frame "ValidateCRC" {
        n128 = xnode ("FIFO Method Node")("Timeout"=0) -> ("Element"=w334:u16, "Timed Out?"=w329:bool)  [unwired: 1 in, 1 out]
        n129 = case shown="False" w329 {
          tunnel: w334 -> [w335 _]
          tunnel: [w343 w345] -> w333
          tunnel: w332 -> [w344 w345]
          tunnel: w331 -> [w338 _]
          frame False {
            n130 = xnode ("Register Read")() -> ("Data"=w337:u64)  [unwired: 1 in, 1 out]
            n131 = Equal?(x=w338, y=w335) -> (x = y?=w342:bool)
            n132 = Select(t=FlowSensorSampleSensorLoopStates."PrepareSample" ("InclinometerState"), s=w342, f=FlowSensorSampleSensorLoopStates."ResponseCRCError" ("InclinometerState")) -> (s? t:f=w339:T2)
            n133 = Increment(x=w337) -> (x+1=w336:u64)
            n134 = xnode ("Register Write")("Data"=w336) -> ()  [unwired: 1 in, 1 out]
            n135 = Bundle By Name(cluster=w344, "State"=w339) -> (w343:T1)
          }
          frame True {
          }
        }
      }
      frame "PrepareSample" {
        n136 = xnode ("Register Read")() -> ("Data"=w349:u64)  [unwired: 1 in, 1 out]
        n137 = xnode ("Register Read")() -> ("Data"=w348:u64)  [unwired: 1 in, 1 out]
        n138 = xnode ("Register Read")() -> ("Data"=w347:u64)  [unwired: 1 in, 1 out]
        n139 = xnode ("Register Read")() -> ("Data"=w346:u64)  [unwired: 1 in, 1 out]
        n140 = Bundle By Name(cluster=w352, "State"=FlowSensorSampleSensorLoopStates."MoveSample", "Sample.Timestamp"=w351, "Sample.TxBytes"=w349, "Sample.RxBytes"=w348, "Sample.TxFrames"=w347, "Sample.RxFrames"=w346) -> (w353:T1)
      }
      frame "MoveSample" {
        n141 = xnode ("FIFO Method Node")("Element"=w354, "Timeout"=0) -> ()  [unwired: 1 in, 2 out]
        n142 = Bundle By Name(cluster=w357, "State"=FlowSensorSampleSensorLoopStates."WaitForTrigger") -> (w358:T1)
      }
      frame "ReadExceptionCode" {
        n143 = xnode ("FIFO Method Node")("Timeout"=0) -> ("Element"=w363:u8, "Timed Out?"=w359:bool)  [unwired: 1 in, 1 out]
        n144 = case shown="False" w359 {
          tunnel: w363 -> [w364 _]
          tunnel: [w375 w377] -> w362
          tunnel: w361 -> [w376 w378]
          frame False {
            n145 = xnode ("FIFO Method Node")("Element"=w364, "Timeout"=0) -> ()  [unwired: 1 in, 2 out]
            n146 = Equal?(x=u8 1, y=w364) -> (x = y?=w368:bool)
            n147 = Equal?(x=u8 2, y=w364) -> (x = y?=w367:bool)
            n148 = Or(x=w368, y=w367) -> (x .or. y?=w366:bool)
            n149 = Select(t=FlowSensorSampleSensorLoopStates."ReadExceptionCRCByte0" ("InclinometerState"), s=w366, f=FlowSensorSampleSensorLoopStates."ResponseUnknownError" ("InclinometerState")) -> (s? t:f=w371:T2)
            n150 = Bundle By Name(cluster=w376, "State"=w371, "Timeout"=0, "Exception"=w364) -> (w375:T1)
          }
          frame True {
            n151 = call "FlowSensorCheckForTimeout.vi"("FlowSensorSampleSensorLoopData in"=w378) -> ("FlowSensorSampleSensorLoopData out"=w377:T1)  [unwired: 10 in]
          }
        }
      }
      frame "ReadExceptionCRCByte0" {
        n152 = xnode ("FIFO Method Node")("Timeout"=0) -> ("Element"=w384:u8, "Timed Out?"=w379:bool)  [unwired: 1 in, 1 out]
        n153 = case shown="False" w379 {
          tunnel: w384 -> [w385 _]
          tunnel: [w395 w397] -> w383
          tunnel: w382 -> [w396 w398]
          tunnel: w381 -> [w387 _]
          frame False {
            n154 = To Unsigned Word Integer(number=w385) -> (unsigned 16bit integer=w389:u16)
            n155 = Logical Shift(y=i16 0, x=w389) -> (x << y=w391:u16)
            n156 = And(x=u16 65280, y=w387) -> (x .and. y?=w390:u16)
            n157 = Or(x=w390, y=w391) -> (x .or. y?=w388:u16)
            n158 = Bundle By Name(cluster=w396, "State"=FlowSensorSampleSensorLoopStates."ReadExceptionCRCByte1" ("InclinometerState"), "CRC"=w388, "Timeout"=0) -> (w395:T1)
          }
          frame True {
            n159 = call "FlowSensorCheckForTimeout.vi"("FlowSensorSampleSensorLoopData in"=w398) -> ("FlowSensorSampleSensorLoopData out"=w397:T1)  [unwired: 10 in]
          }
        }
      }
      frame "ReadExceptionCRCByte1" {
        n160 = xnode ("FIFO Method Node")("Timeout"=0) -> ("Element"=w404:u8, "Timed Out?"=w399:bool)  [unwired: 1 in, 1 out]
        n161 = case shown="False" w399 {
          tunnel: w404 -> [w405 _]
          tunnel: [w415 w417] -> w403
          tunnel: w402 -> [w416 w418]
          tunnel: w401 -> [w407 _]
          frame False {
            n162 = To Unsigned Word Integer(number=w405) -> (unsigned 16bit integer=w409:u16)
            n163 = Logical Shift(y=i16 8, x=w409) -> (x << y=w411:u16)
            n164 = And(x=u16 255, y=w407) -> (x .and. y?=w410:u16)
            n165 = Or(x=w410, y=w411) -> (x .or. y?=w408:u16)
            n166 = Bundle By Name(cluster=w416, "State"=FlowSensorSampleSensorLoopStates."CalculateExceptionCRC" ("InclinometerState"), "CRC"=w408, "Timeout"=0) -> (w415:T1)
          }
          frame True {
            n167 = call "FlowSensorCheckForTimeout.vi"("FlowSensorSampleSensorLoopData in"=w418) -> ("FlowSensorSampleSensorLoopData out"=w417:T1)  [unwired: 10 in]
          }
        }
      }
      frame "CalculateExceptionCRC" {
        n168 = xnode ("FIFO Method Node")("Element"=TRUE, "Timeout"=0) -> ()  [unwired: 1 in, 2 out]
        n169 = Bundle By Name(cluster=w422, "State"=FlowSensorSampleSensorLoopStates."ValidateExceptionCRC" ("InclinometerState")) -> (w423:T1)
      }
      frame "ValidateExceptionCRC" {
        n170 = xnode ("FIFO Method Node")("Timeout"=0) -> ("Element"=w429:u16, "Timed Out?"=w424:bool)  [unwired: 1 in, 1 out]
        n171 = case shown="False" w424 {
          tunnel: w429 -> [w430 _]
          tunnel: [w438 w440] -> w428
          tunnel: w427 -> [w439 w440]
          tunnel: w426 -> [w433 _]
          frame False {
            n172 = xnode ("Register Read")() -> ("Data"=w432:u64)  [unwired: 1 in, 1 out]
            n173 = Equal?(x=w433, y=w430) -> (x = y?=w437:bool)
            n174 = Select(t=FlowSensorSampleSensorLoopStates."ParseExceptionCode" ("InclinometerState"), s=w437, f=FlowSensorSampleSensorLoopStates."ResponseCRCError" ("InclinometerState")) -> (s? t:f=w434:T2)
            n175 = Increment(x=w432) -> (x+1=w431:u64)
            n176 = xnode ("Register Write")("Data"=w431) -> ()  [unwired: 1 in, 1 out]
            n177 = Bundle By Name(cluster=w439, "State"=w434) -> (w438:T1)
          }
          frame True {
          }
        }
      }
      frame "ParseExceptionCode" {
        n178 = Equal?(x=w442, y=u8 1) -> (x = y?=w446:bool)
        n179 = Select(t=FlowSensorSampleSensorLoopStates."SensorReportsIllegalFunction" ("InclinometerState"), s=w446, f=FlowSensorSampleSensorLoopStates."SensorReportsIllegalDataAddress" ("InclinometerState")) -> (s? t:f=w443:T2)
        n180 = Bundle By Name(cluster=w447, "State"=w443) -> (w448:T1)
      }
      frame "ResponseAddressError" {
        n181 = Bundle By Name(cluster=w451, "State"=FlowSensorSampleSensorLoopStates."PrepareErrorCode" ("InclinometerState"), "ErrorSample.ErrorCode"=FlowSensorErrorCodes."ResponseAddressError" ("InclinometerErrorCodes")) -> (w452:T1)
      }
      frame "ResponseFunctionCodeError" {
        n182 = Bundle By Name(cluster=w455, "State"=FlowSensorSampleSensorLoopStates."PrepareErrorCode" ("InclinometerState"), "ErrorSample.ErrorCode"=FlowSensorErrorCodes."ResponseFunctionCodeError" ("InclinometerErrorCodes")) -> (w456:T1)
      }
      frame "ResponseByteCountError" {
        n183 = Bundle By Name(cluster=w459, "State"=FlowSensorSampleSensorLoopStates."PrepareErrorCode" ("InclinometerState"), "ErrorSample.ErrorCode"=FlowSensorErrorCodes."ResponseByteCountError" ("InclinometerErrorCodes")) -> (w460:T1)
      }
      frame "ResponseCRCError" {
        n184 = Bundle By Name(cluster=w463, "State"=FlowSensorSampleSensorLoopStates."PrepareErrorCode" ("InclinometerState"), "ErrorSample.ErrorCode"=FlowSensorErrorCodes."ResponseCRCError" ("InclinometerErrorCodes")) -> (w464:T1)
      }
      frame "ResponseUnknownError" {
        n185 = Bundle By Name(cluster=w467, "State"=FlowSensorSampleSensorLoopStates."PrepareErrorCode" ("InclinometerState"), "ErrorSample.ErrorCode"=FlowSensorErrorCodes."ResponseUnknownError" ("InclinometerErrorCodes")) -> (w468:T1)
      }
      frame "ResponseTimeoutError" {
        n186 = Bundle By Name(cluster=w471, "State"=FlowSensorSampleSensorLoopStates."PrepareErrorCode" ("InclinometerState"), "ErrorSample.ErrorCode"=FlowSensorErrorCodes."ResponseTimeoutError" ("InclinometerErrorCodes")) -> (w472:T1)
      }
      frame "SensorReportsIllegalFunction" {
        n187 = Bundle By Name(cluster=w475, "State"=FlowSensorSampleSensorLoopStates."PrepareErrorCode" ("InclinometerState"), "ErrorSample.ErrorCode"=FlowSensorErrorCodes."SensorReportsIllegalFunction" ("InclinometerErrorCodes")) -> (w476:T1)
      }
      frame "SensorReportsIllegalDataAddress" {
        n188 = Bundle By Name(cluster=w479, "State"=FlowSensorSampleSensorLoopStates."PrepareErrorCode" ("InclinometerState"), "ErrorSample.ErrorCode"=FlowSensorErrorCodes."SensorReportsIllegalDataAddress" ("InclinometerErrorCodes")) -> (w480:T1)
      }
      frame "PrepareErrorCode" {
        n189 = xnode ("Register Read")() -> ("Data"=w484:u64)  [unwired: 1 in, 1 out]
        n190 = xnode ("Register Read")() -> ("Data"=w483:u64)  [unwired: 1 in, 1 out]
        n191 = xnode ("Register Read")() -> ("Data"=w482:u64)  [unwired: 1 in, 1 out]
        n192 = xnode ("Register Read")() -> ("Data"=w481:u64)  [unwired: 1 in, 1 out]
        n193 = Bundle By Name(cluster=w487, "State"=FlowSensorSampleSensorLoopStates."MoveErrorCode", "ErrorSample.Timestamp"=w486, "ErrorSample.TxBytes"=w484, "ErrorSample.RxBytes"=w483, "ErrorSample.TxFrames"=w482, "ErrorSample.RxFrames"=w481) -> (w488:T1)
      }
      frame "MoveErrorCode" {
        n194 = xnode ("FIFO Method Node")("Element"=w490, "Timeout"=0) -> ()  [unwired: 1 in, 2 out]
        n195 = Bundle By Name(cluster=w492, "State"=FlowSensorSampleSensorLoopStates."WaitForTrigger") -> (w493:T1)
      }
    }
  }
  n196 = node-c288(w2) -> ()
